vi "Get File Paths and Versions.vi"(7 "relative paths? (F: Absolute)":bool, 8 "error in (no error)":errorcluster, 11 "Session in":refnum<class "Session.lvclass">) -> (0 "error out":errorcluster, 1 "Versions":string[](array[string]), 2 "File Paths":path[](array[path]), 3 "Session out":refnum<class "Session.lvclass">)   [LabVIEW 2020, in "Save for Previous Version.lvlib" / "Session.lvclass"]
uses:
  Session.lvclass
  Session.lvclass/Session.ctl
  LabVIEW File/LabVIEW File.lvclass
  File/File.lvclass/File.lvclass
  <userlib>/_OpenG.lib/file/file.llb/Compare Two Paths - Path2 Array__ogtk.vi
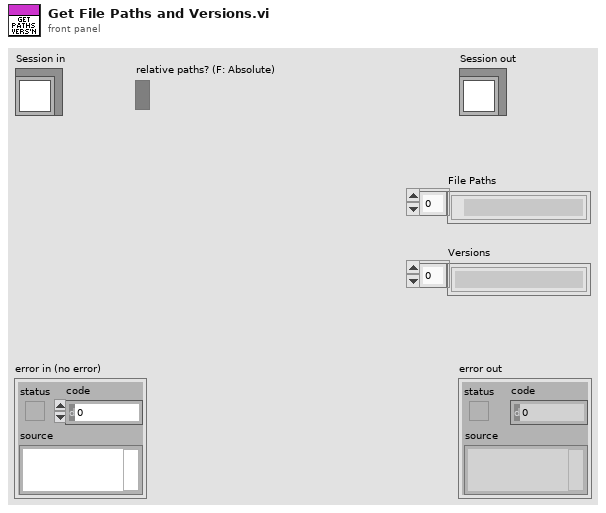
[diagram p1: front panel]
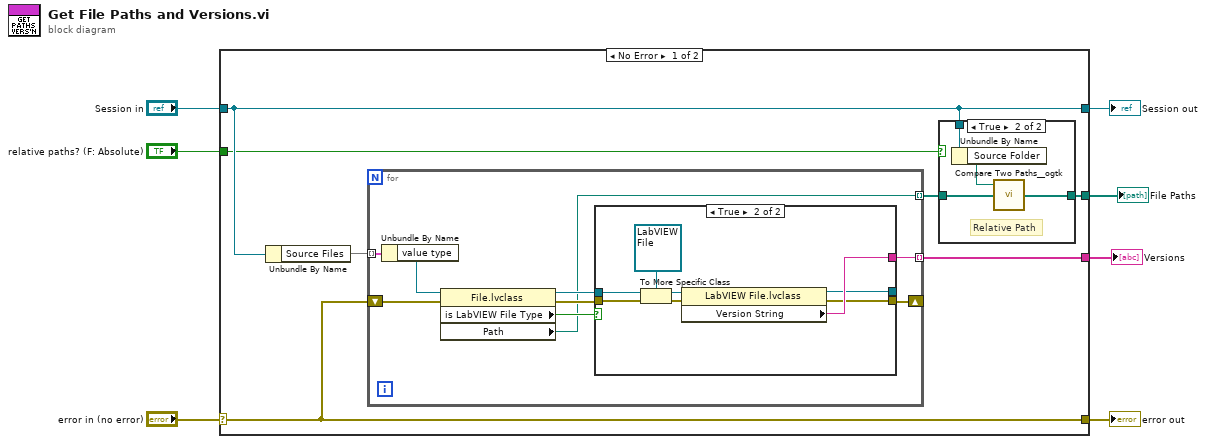
[diagram p0: block diagram]
diagram:
  n1 = case shown="No Error" "error in (no error)" {
    selector: "error in (no error)" -> [w13 w39]
    tunnel: [w13 w39] -> w6
    tunnel: [w11 w38] -> w4
    tunnel: "Session in" -> [w11 w38]
    tunnel: [w12 _] -> w3
    tunnel: [w9 _] -> w2
    tunnel: "relative paths? (F: Absolute)" -> [w8 _]
    frame No Error {
      n2 = Unbundle By Name(w11) -> ("Source Files"=w14:map{path, refnum<class "File.lvclass">})
      n3 = for {
        tunnel: w14 -> [w26] mode=indexing
        shift-right: [w23] -> _
        shift-left: w13 -> [w24]
        tunnel: [w22] -> w12 mode=indexing
        tunnel: [w21] -> w10 mode=indexing
        n4 = Unbundle By Name(w26) -> ("value type"=w20:refnum<class "File.lvclass">)
        n5 = property class="File.lvclass"(reference=w20, error in=w24) -> (reference out=w27:refnum<class "File.lvclass">, error out=w25:errorcluster, "is LabVIEW File Type"=w28:bool, "Path"=w21:path)
        n6 = case shown="True" w28 {
          tunnel: w27 -> [_ w36]
          tunnel: [_ w34] -> w22
          tunnel: [w29 w33] -> w23
          tunnel: w25 -> [w29 w31]
          tunnel: [_ w30] -> _
          frame False {
          }
          frame True {
            n7 = To More Specific Class(target class=refnum<class "LabVIEW File.lvclass"> refnum ("Save for Previous Version.lvlib:LabVIEW File.lvclass"), reference=w36, error in=w31) -> (specific class reference=w35:refnum<class "LabVIEW File.lvclass">, error out=w32:errorcluster)
            n8 = property class="LabVIEW File.lvclass"(reference=w35, error in=w32) -> (reference out=w30:refnum<class "LabVIEW File.lvclass">, error out=w33:errorcluster, "Version String"=w34:string)
          }
        }
      }
      n9 = case shown="True" w8 {
        tunnel: w11 -> [_ w19]
        tunnel: w10 -> [w15 w17]
        tunnel: [w15 w16] -> w9
        frame False {
        }
        frame True {
          # "Relative Path"
          n10 = Unbundle By Name(w19) -> ("Source Folder"=w18:path)
          n11 = call-poly <userlib>:"Compare Two Paths__ogtk.vi"("path2"=w17, "path1"=w18) -> ("relative path from 1 to 2"=w16:path[])  [unwired: 1 in, 2 out]
        }
      }
    }
    frame Error {
    }
  }
  "error out" <- w6
  "Session out" <- w4
  "File Paths" <- w2
  "Versions" <- w3
